vi "test-NameMap.vi"(8 "error in (no error)":errorcluster, 11 "TestCase in":refnum<class "MyTestCase.lvclass">) -> (0 "error out":errorcluster, 3 "TestCase out":refnum<class "MyTestCase.lvclass">)   [LabVIEW 2019, in "MyTestCase.lvclass"]
uses:
  MyTestCase.lvclass
  <vilib>/addons/_JKI Toolkits/VI Tester/TestCase.llb/TestCase.lvclass
  src/lv-apt-json-file.lvlib
  C:/Program Files (x86)/National Instruments/LabVIEW 2019/vi.lib/addons/_JKI Toolkits/VI Tester/TestCase.llb/TestCase.lvclass
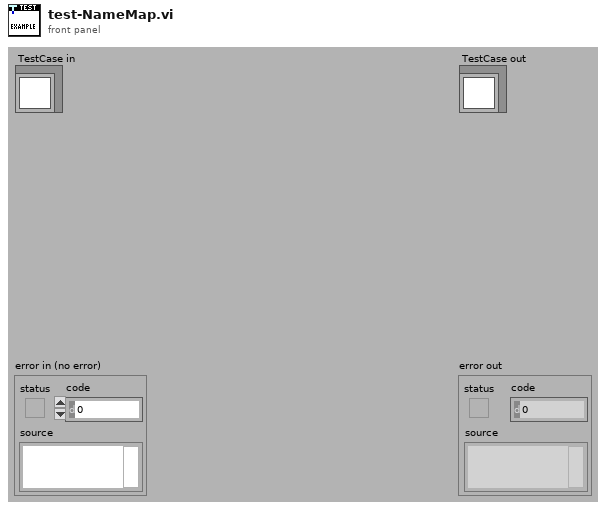
[diagram p1: front panel]
types:
  T1 = typedef "lv-apt-json-file.lvlib/Def-NameMap.ctl" = variant[]
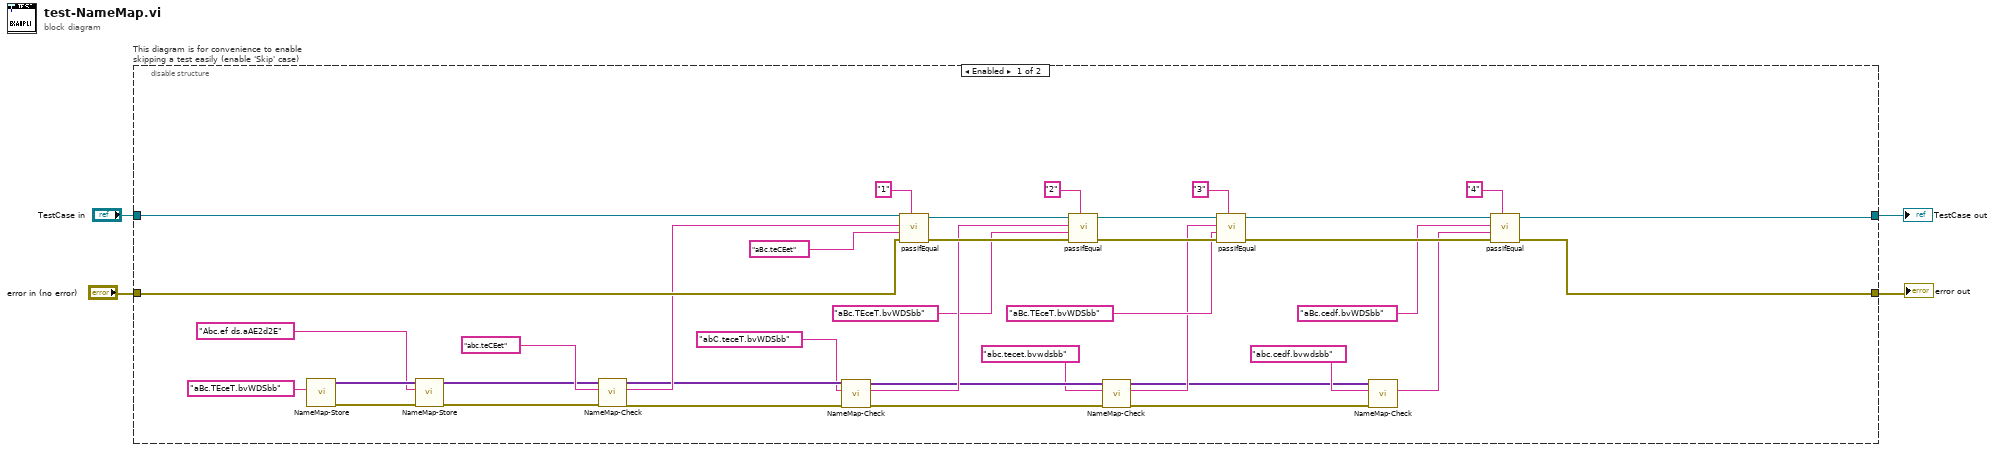
[diagram p0: block diagram]
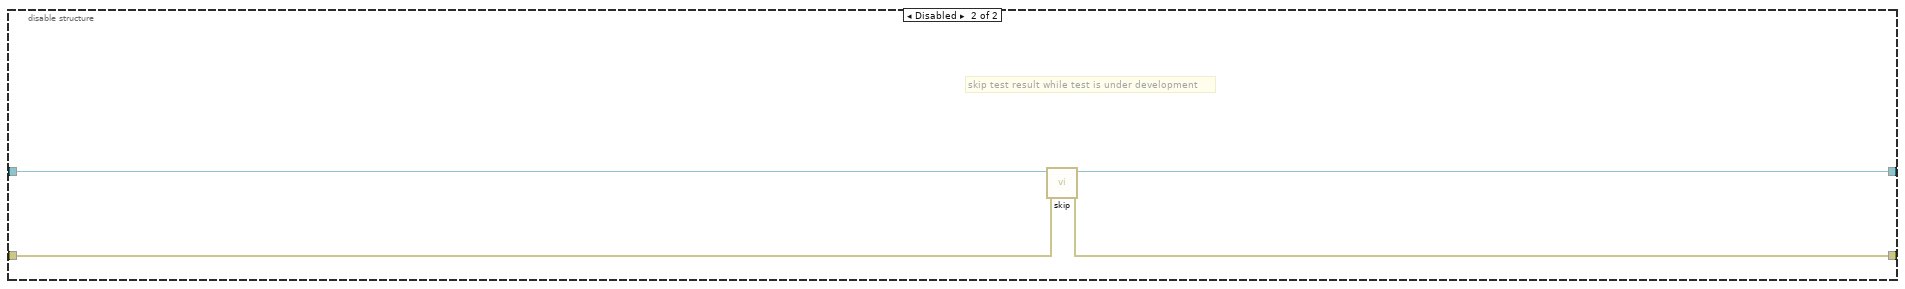
[diagram p2: hidden frame]
diagram:
  n1 = disable-structure "This diagram is for convenience to enable skipping a test easily (enable 'Skip' case)" shown="Enabled" {
    disable-tunnel: "TestCase in" -> [w31 w46]
    disable-tunnel: [w17 w44] -> w1
    disable-tunnel: [w15 w45] -> w3
    disable-tunnel: "error in (no error)" -> [w30 w43]
    frame Enabled {
      n2 = call "NameMap-Store.vi"("name"="aBc.TEceT.bvWDSbb") -> ("error out"=w40:errorcluster, "NameMap out"=w39:T1)  [unwired: 9 in]
      n3 = call "NameMap-Store.vi"("error in (no error)"=w40, "name"="Abc.ef ds.aAE2d2E", "NameMap in"=w39) -> ("error out"=w37:errorcluster, "NameMap out"=w38:T1)  [unwired: 7 in]
      n4 = call "NameMap-Check.vi"("error in (no error)"=w37, "Name"="abc.teCEet", "NameMap in"=w38) -> ("error out"=w26:errorcluster, "OriginName"=w29:string, "NameMap out"=w27:T1)  [unwired: 6 in]
      n5 = call "NameMap-Check.vi"("error in (no error)"=w26, "Name"="abC.teceT.bvWDSbb" ("name"), "NameMap in"=w27) -> ("error out"=w11:errorcluster, "OriginName"=w25:string, "NameMap out"=w21:T1)  [unwired: 6 in]
      n6 = call-dynamic "passIfEqual.vi"("custom report message (\"\")"="1" ("custom report message (\"\")"), "error in (no error)"=w30, "y"="aBc.teCEet" ("Name"), "x"=w29, "TestCase in"=w31) -> ("error out"=w34:errorcluster, "TestCase out"=w35:refnum<class "MyTestCase.lvclass">)  [unwired: 5 in]
      n7 = call-dynamic "passIfEqual.vi"("custom report message (\"\")"="2" ("custom report message (\"\")"), "error in (no error)"=w34, "y"="aBc.TEceT.bvWDSbb" ("name"), "x"=w25, "TestCase in"=w35) -> ("error out"=w32:errorcluster, "TestCase out"=w33:refnum<class "MyTestCase.lvclass">)  [unwired: 5 in]
      n8 = call "NameMap-Check.vi"("error in (no error)"=w11, "Name"="abc.tecet.bvwdsbb" ("name"), "NameMap in"=w21) -> ("error out"=w12:errorcluster, "OriginName"=w19:string, "NameMap out"=w13:T1)  [unwired: 6 in]
      n9 = call-dynamic "passIfEqual.vi"("custom report message (\"\")"="3" ("custom report message (\"\")"), "error in (no error)"=w32, "y"="aBc.TEceT.bvWDSbb" ("name"), "x"=w19, "TestCase in"=w33) -> ("error out"=w16:errorcluster, "TestCase out"=w18:refnum<class "MyTestCase.lvclass">)  [unwired: 5 in]
      n10 = call "NameMap-Check.vi"("error in (no error)"=w12, "Name"="abc.cedf.bvwdsbb" ("name"), "NameMap in"=w13) -> ("OriginName"=w10:string)  [unwired: 6 in, 2 out]
      n11 = call-dynamic "passIfEqual.vi"("custom report message (\"\")"="4" ("custom report message (\"\")"), "error in (no error)"=w16, "y"=w10, "x"="aBc.cedf.bvWDSbb" ("name"), "TestCase in"=w18) -> ("error out"=w15:errorcluster, "TestCase out"=w17:refnum<class "MyTestCase.lvclass">)  [unwired: 5 in]
    }
    frame Disabled {
      # "skip test result while test is under development"
      n12 = call <vilib>:"skip.vi"("error in (no error)"=w43, "TestCase in"=w46) -> ("error out"=w45:errorcluster, "TestCase out"=w44:refnum<class "MyTestCase.lvclass">)  [unwired: 8 in]
    }
  }
  "error out" <- w3
  "TestCase out" <- w1
